vi "Perform Action.vi"(8 "error in (no error)":errorcluster, 10 "Input":variant, 11 "DIO DAQmx PWM CFG in":refnum<class "DIO DAQmx PWM CFG.lvclass">) -> (0 "error out":errorcluster, 2 "Output":variant, 3 "DIO DAQmx PWM CFG out":refnum<class "DIO DAQmx PWM CFG.lvclass">)   [LabVIEW 2023, in "DIO DAQmx PWM CFG.lvclass"]
uses:
  DIO DAQmx PWM CFG.lvclass
  D:/git/HAL/HAL GOOP4/DAQmx/DAQmx Base CFG/DAQmx Base CFG.lvclass
  DAQmx/DAQmx Base CFG/DAQmx Base CFG.lvclass/DAQmx Base CFG.ctl
  DIO DAQmx PWM CFG.lvclass/DIO DAQmx PWM CFG.ctl
  DAQmx/DAQmx Base CFG/DAQmx Base CFG.lvclass
  <resource>/objmgr/daqmx.rc
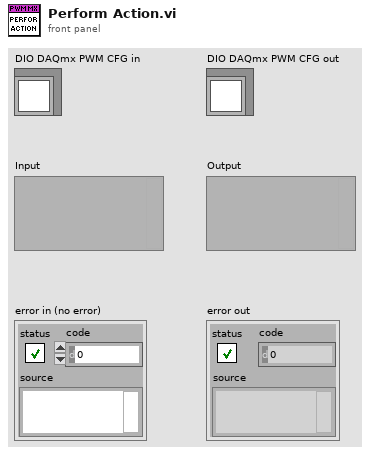
[diagram p1: front panel]
types:
  T1 = cluster{"Channel":string, "PWM Pams":cluster{"Frequency":dbl, "Duty Cycle":dbl}}
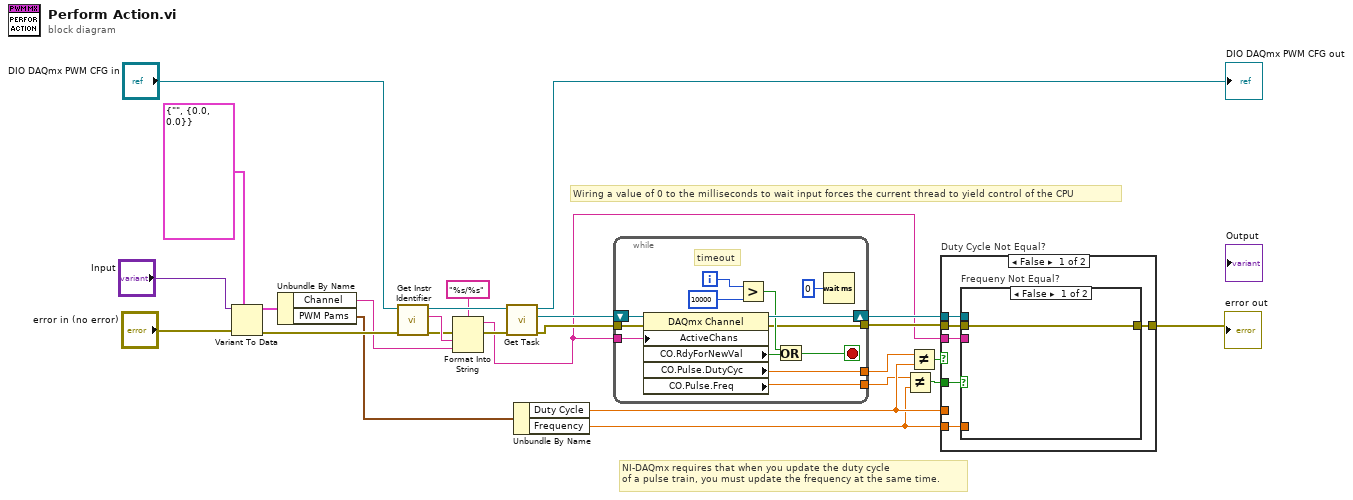
[diagram p0: block diagram]
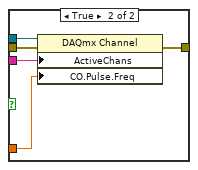
[diagram p2: hidden frame]
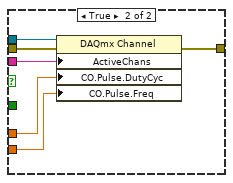
[diagram p3: hidden frame]
diagram:
  # "Wiring a value of 0 to the milliseconds to wait input forces the current thread to yield control of the CPU"
  # "NI-DAQmx requires that when you update the duty cycle\nof a pulse train, you must update the frequency at the same time."
  n1 = Variant To Data(error in="error in (no error)", type=T1 {"Channel"="", "PWM Pams"={"Frequency"=0.0, "Duty Cycle"=0.0}}, Variant="Input") -> (data=w21:T1, error out=w22:errorcluster)
  n2 = Unbundle By Name(w21) -> ("Channel"=w15:string, "PWM Pams"=w12:cluster{"Frequency":dbl, "Duty Cycle":dbl})
  n3 = call-dynamic "Get Instr Identifier.vi"("error in (no error)"=w22, "Configuration Base in"="DIO DAQmx PWM CFG in") -> ("error out"=w14:errorcluster, "Instr Identifier"=w16:string, "Configuration Base out"=w19:refnum<class "DIO DAQmx PWM CFG.lvclass">)  [unwired: 7 in]
  n4 = Format Into String(format string="%s/%s", error in=w14, w16, w15) -> (resulting string=w1:string, error out=w13:errorcluster)  [unwired: 1 in]
  n5 = call "Get Task.vi"("error in (no error)"=w13, "DAQmx Base CFG in"=w19) -> ("error out"=w5:errorcluster, "Task"=w4:refnum<k21>, "DAQmx Base CFG out"=→"DIO DAQmx PWM CFG out":refnum<class "DIO DAQmx PWM CFG.lvclass">)  [unwired: 7 in]
  n6 = Unbundle By Name(w12) -> ("Duty Cycle"=w10:dbl, "Frequency"=w6:dbl)
  n7 = while {
    tunnel: [w38] -> w9
    tunnel: w5 -> [w37]
    tunnel: [w35] -> w3
    tunnel: w1 -> [w34]
    shift-right: [w39] -> w11
    shift-left: w4 -> [w36]
    tunnel: [w27] -> w2
    i -> [w32]
    stop <- w30 stop-if-true
    # "timeout"
    n8 = property class="DAQmx Channel"(reference=w36, error in=w37, "ActiveChans"=w34) -> (reference out=w39:refnum<k21>, error out=w27:errorcluster, "CO.RdyForNewVal"=w33:bool, "CO.Pulse.DutyCyc"=w38:dbl, "CO.Pulse.Freq"=w35:dbl)
    n9 = Greater?(x=w32, y=10000) -> (0:w29:bool)
    n10 = Or(x=w29, y=w33) -> (x .or. y?=w30:bool)
    n11 = Wait (ms)(milliseconds to wait=u32 0) -> ()  [unwired: 1 out]
  }
  n12 = Not Equal?(x=w3, y=w6) -> (x != y?=w7:bool)
  n13 = Not Equal?(x=w9, y=w10) -> (x != y?=w8:bool)
  n14 = case "Duty Cycle Not Equal?" shown="False" w8 {
    tunnel: [w42 w57] -> w18
    tunnel: w6 -> [w43 w56]
    tunnel: w2 -> [w45 w55]
    tunnel: w11 -> [w41 w54]
    tunnel: w10 -> [_ w53]
    tunnel: w7 -> [w44 _]
    tunnel: w1 -> [w40 w52]
    frame False {
      n15 = case "Frequeny Not Equal?" shown="False" w44 {
        tunnel: w45 -> [w46 w51]
        tunnel: w43 -> [_ w48]
        tunnel: [w46 w50] -> w42
        tunnel: w41 -> [_ w49]
        tunnel: w40 -> [_ w47]
        frame False {
        }
        frame True {
          n16 = property class="DAQmx Channel"(reference=w49, error in=w51, "ActiveChans"=w47, "CO.Pulse.Freq"=w48) -> (error out=w50:errorcluster)  [unwired: 1 out]
        }
      }
    }
    frame True {
      n17 = property class="DAQmx Channel"(reference=w54, error in=w55, "ActiveChans"=w52, "CO.Pulse.DutyCyc"=w53, "CO.Pulse.Freq"=w56) -> (error out=w57:errorcluster)  [unwired: 1 out]
    }
  }
  "error out" <- w18
